vi "displayLineByLine.vi"(8 "error in (no error)":errorcluster, 10 "scoreLog":string[][](table), 11 "TextDisplay Class in":refnum<class "TextDisplay Class.lvclass">) -> (0 "error out":errorcluster, 3 "TextDisplay Class out":refnum<class "TextDisplay Class.lvclass">)   [LabVIEW 2019, in "TextDisplay Class.lvclass"]
uses:
  TextDisplay Class.lvclass
  TextDisplay Class.lvclass/TextDisplay Class.ctl
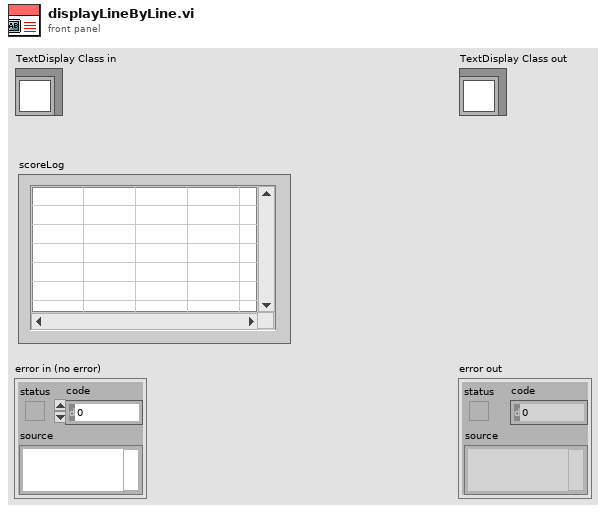
[diagram p1: front panel]
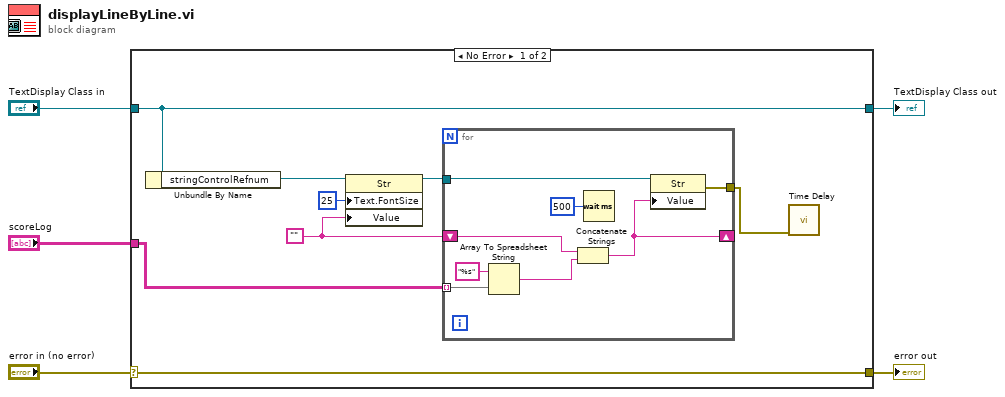
[diagram p0: block diagram]
diagram:
  n1 = case shown="No Error" "error in (no error)" {
    selector: "error in (no error)" -> [w13 w23]
    tunnel: [w13 w23] -> w4
    tunnel: [w11 w22] -> w2
    tunnel: "TextDisplay Class in" -> [w11 w22]
    tunnel: "scoreLog" -> [w12 _]
    frame No Error {
      w7 = ""
      n2 = Unbundle By Name(w11) -> ("stringControlRefnum"=w8:refnum<vi>)
      n3 = property class="Str"(reference=w8, "Text.FontSize"=u32 25 ("Text.Font:Size"), "Value"=w7) -> (reference out=w9:refnum<vi>)  [unwired: 1 in, 1 out]
      n4 = for {
        shift-right: [w15] -> _
        shift-left: w7 -> [w18]
        tunnel: w12 -> [w20] mode=indexing
        tunnel: w9 -> [w16]
        tunnel: [w14] -> w6
        n5 = Array To Spreadsheet String(array=w20, 3:"%s" ("format string")) -> (spreadsheet string=w17:string)  [unwired: 1 in]
        n6 = Concatenate Strings(w18, w17) -> (w15:string)
        n7 = Wait (ms)(milliseconds to wait=u32 500) -> ()  [unwired: 1 out]
        n8 = property class="Str"(reference=w16, "Value"=w15) -> (error out=w14:errorcluster)  [unwired: 1 in, 1 out]
      }
      n9 = call "Time Delay"("error in (no error)"=w6) -> ()  [unwired: 10 in, 1 out]
    }
    frame Error {
    }
  }
  "error out" <- w4
  "TextDisplay Class out" <- w2
